vi "手绘波形子VI.vi"() -> (0 "输出的波形":waveform(dbl)(graph), 1 "最小值":dbl format="%#_3g", 2 "最大值":dbl format="%#_3g", 3 "频率":dbl)   [LabVIEW 2017]
uses:
  <vilib>/gmath/NI_Gmath.lvlib
panel:
  in  "选项卡控件":enum32{"手绘和参数设置", "输出的波形图", "使用说明"}(tab)
  out "绘 图 区":cluster{dbl, dbl}[](graph)
  in  "绘图完成":bool
  in  "时间长度":dbl=0.1
  in  "幅值":dbl=1.0
  # "手 绘 波 形"
  # "s"
  # "Hz"
  # "说明：\n1、鼠标在画板上单击并从左到右拖动，绘出所需的波形图；\n2、鼠标松开，鼠标单击绘图完成，自动生成所绘制的波形并退出此绘图界面；\n3、如果在上述绘图过程中，想重新绘制，可以点击幅值或者时间长度\n，只要其值发生改变，绘图区会自动清零."
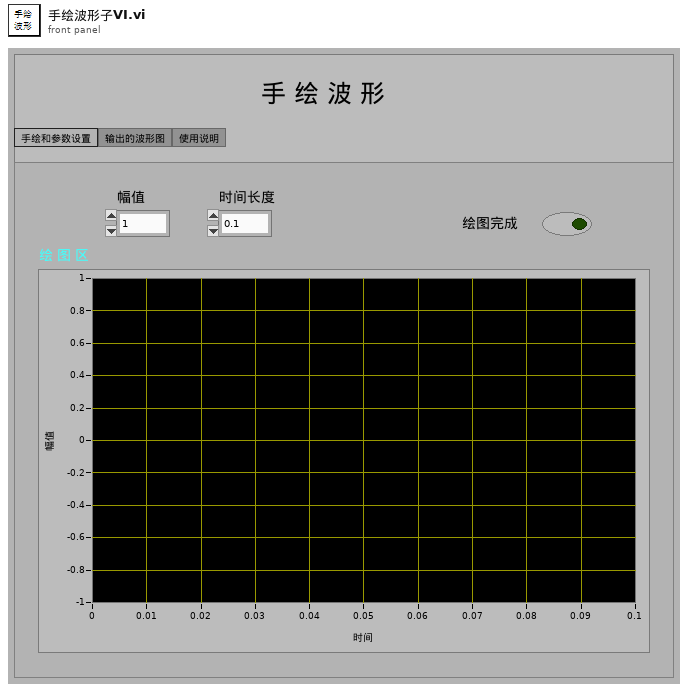
[diagram p1: front panel]
types:
  T1 = enum8{"Enabled", "Disabled", "Disabled and Grayed Out"}
  T2 = typedef "LVPoint32TypeDef.ctl" = cluster{"Horizontal":i32, "Vertical":i32}
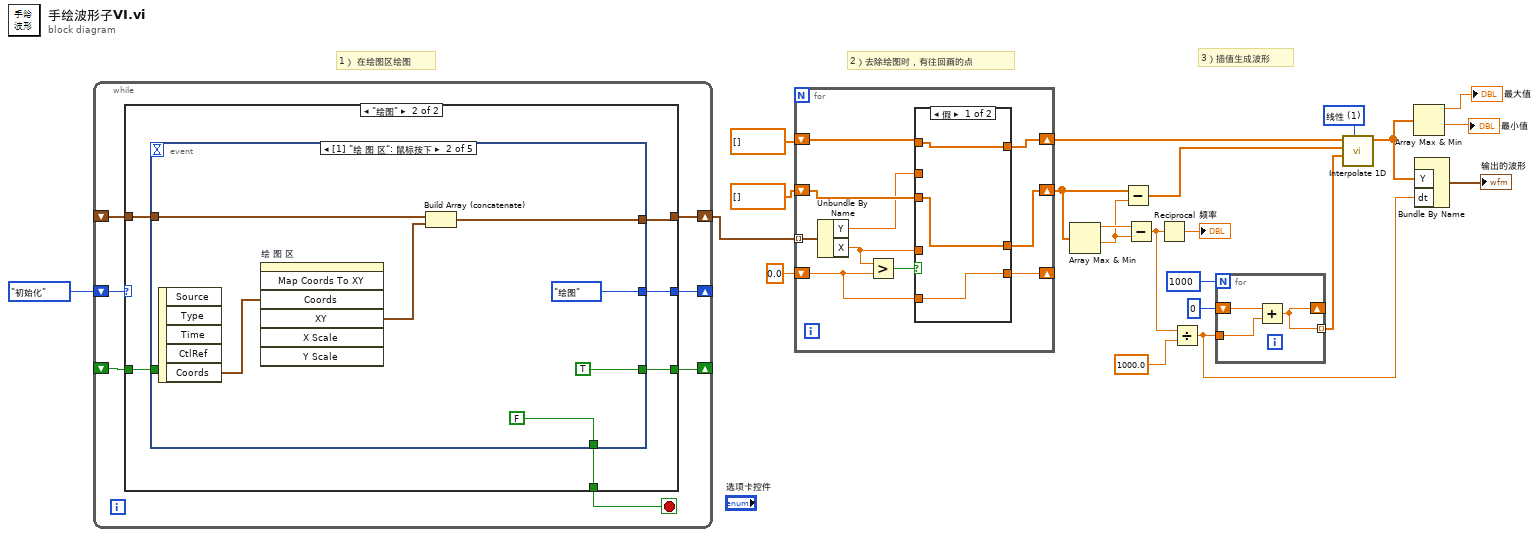
[diagram p0: block diagram]
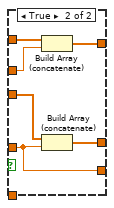
[diagram p2: hidden frame]
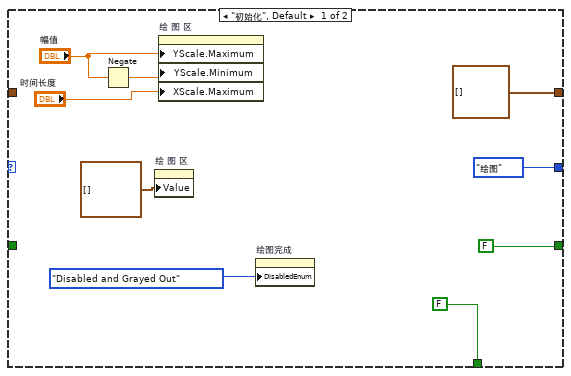
[diagram p3: hidden frame]
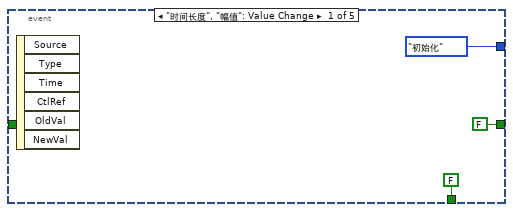
[diagram p4: hidden frame]
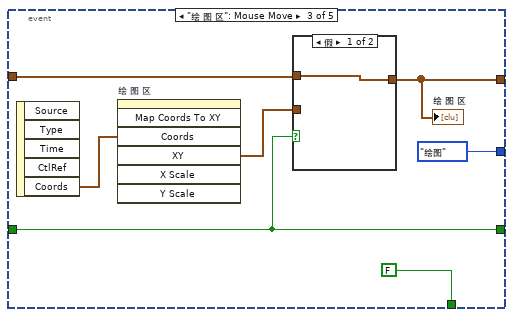
[diagram p5: hidden frame]
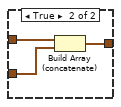
[diagram p6: hidden frame]
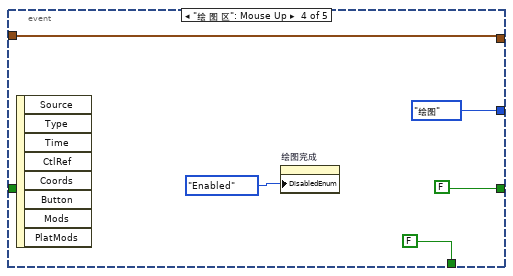
[diagram p7: hidden frame]
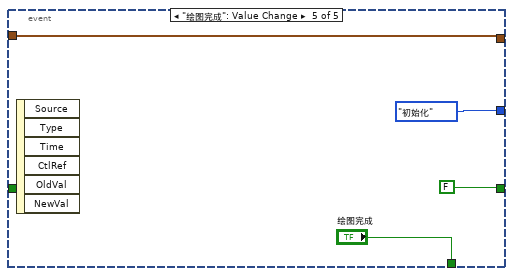
[diagram p8: hidden frame]
diagram:
  w14 = 1 items=["最近", "线性", "样条", "cubic Hermite", "拉格朗日"] ("method")
  # "3）插值生成波形"
  # "2）去除绘图时，有往回画的点"
  # "1） 在绘图区绘图"
  n1 = while {
    shift-right: [w29] -> w22
    shift-left: _ -> [w28]
    shift-right: [w23] -> _
    shift-left: enum16{"初始化", "绘图"}."初始化" -> [w27]
    shift-right: [w26] -> _
    shift-left: _ -> [w25]
    stop <- w24 stop-if-true
    n2 = case shown="\"绘图\"" w27 {
      tunnel: [cluster{"X":dbl, "Y":dbl}[] [] w44] -> w29
      tunnel: w28 -> [_ w43]
      tunnel: [FALSE ("press") w42] -> w26
      tunnel: w25 -> [_ w41]
      tunnel: [FALSE w40] -> w24
      tunnel: [enum16{"初始化", "绘图"}."绘图" w39] -> w23
      frame "初始化", Default {
        n3 = Negate(x="幅值") -> (-x=w37:dbl)
        n4 = property on="绘 图 区" class="XYGraph (严格)"("Value"=cluster{dbl, dbl}[] [] ("绘 图 区")) -> ()  [unwired: 2 in, 2 out]
        n5 = property on="绘 图 区" class="XYGraph (严格)"("YScale.Maximum"="幅值", "YScale.Minimum"=w37, "XScale.Maximum"="时间长度") -> ()  [unwired: 2 in, 2 out]
        n6 = property on="绘图完成" class="Bool"("DisabledEnum"=T1."Disabled and Grayed Out" ("禁用")) -> ()  [unwired: 2 in, 2 out]
      }
      frame "绘图" {
        n7 = event shown="[1] \"绘 图 区\": 鼠标按下" {
          selector: _ -> [_ _ _ _ _]
          dyn-events: _ -> [_ _ _ _ _]
          timeout: _ -> [_ _ _ _ _]
          tunnel: w43 -> [_ w53 w60 w70 w73]
          tunnel: [_ w51 w58 w70 w73] -> w44
          tunnel: [FALSE ("press") TRUE ("press") w57 FALSE ("press") FALSE ("press")] -> w42
          tunnel: w41 -> [_ _ w57 _ _]
          tunnel: [FALSE ("绘图完成") FALSE FALSE FALSE "绘图完成"] -> w40
          tunnel: [enum16{"初始化", "绘图"}."初始化" enum16{"初始化", "绘图"}."绘图" enum16{"初始化", "绘图"}."绘图" enum16{"初始化", "绘图"}."绘图" enum16{"初始化", "绘图"}."初始化"] -> w39
          event "时间长度", "幅值": Value Change {
            n8 = event-data() -> ()  [unwired: 1 in, 6 out]
          }
          event "绘 图 区": Mouse Down {
            n9 = event-data() -> ("Coords"=w54:T2)  [unwired: 1 in, 4 out]
            n10 = invoke on="绘 图 区" class="XYGraph (严格)" method="Map Coords To XY"("Coords"=w54) -> ("XY"=w52:cluster{"X":dbl, "Y":dbl})  [unwired: 6 in, 6 out]
            n11 = Build Array (concatenate)(w53, w52) -> (w51:cluster{"X":dbl, "Y":dbl}[])
          }
          event "绘 图 区": Mouse Move {
            n12 = event-data() -> ("Coords"=w61:T2)  [unwired: 1 in, 4 out]
            n13 = invoke on="绘 图 区" class="XYGraph (严格)" method="Map Coords To XY"("Coords"=w61) -> ("XY"=w59:cluster{"X":dbl, "Y":dbl})  [unwired: 6 in, 6 out]
            n14 = case shown="假" w57 {
              tunnel: w60 -> [w62 w65]
              tunnel: w59 -> [_ w64]
              tunnel: [w62 w63] -> w58
              frame False {
              }
              frame True {
                n15 = Build Array (concatenate)(w65, w64) -> (w63:cluster{"X":dbl, "Y":dbl}[])
              }
            }
            "绘 图 区" <- w58
          }
          event "绘 图 区": Mouse Up {
            n16 = event-data() -> ()  [unwired: 1 in, 8 out]
            n17 = property on="绘图完成" class="Bool"("DisabledEnum"=T1."Enabled" ("禁用")) -> ()  [unwired: 2 in, 2 out]
          }
          event "绘图完成": Value Change {
            n18 = event-data() -> ()  [unwired: 1 in, 6 out]
          }
        }
      }
    }
  }
  n19 = for {
    tunnel: w22 -> [w83] mode=indexing
    shift-right: [w80] -> w8
    shift-left: dbl[] [] -> [w82]
    shift-right: [w81] -> w2
    shift-left: dbl[] [] -> [w78]
    shift-right: [w79] -> _
    shift-left: 0.0 ("X") -> [w75]
    n20 = Unbundle By Name(w83) -> ("Y"=w76:dbl, "X"=w77:dbl)
    n21 = Greater?(x=w77, y=w75) -> (0:w84:bool)
    n22 = case shown="假" w84 {
      tunnel: w77 -> [_ w88]
      tunnel: w82 -> [w86 w90]
      tunnel: w76 -> [_ w91]
      tunnel: w78 -> [w87 w93]
      tunnel: [w87 w92] -> w81
      tunnel: [w86 w89] -> w80
      tunnel: [w85 w88] -> w79
      tunnel: w75 -> [w85 _]
      frame False {
      }
      frame True {
        n23 = Build Array (concatenate)(w93, w91) -> (w92:dbl[])
        n24 = Build Array (concatenate)(w90, w88) -> (w89:dbl[])
      }
    }
  }
  n25 = Array Max & Min(array=w8) -> (max value=w10:dbl, min value=w9:dbl)  [unwired: 2 out]
  n26 = Subtract(x=w8, y=w9) -> (x-y=w5:dbl[])
  n27 = Subtract(x=w10, y=w9) -> (x-y=w4:dbl)
  n28 = Reciprocal(x=w4) -> (1/x=→"频率":dbl)
  n29 = Divide(x=w4, y=1000.0) -> (x/y=w3:dbl)
  n30 = for {
    N: 1000 -> [_]
    shift-right: [w94] -> _
    shift-left: 0 -> [w95]
    tunnel: w3 -> [w96]
    tunnel: [w94] -> w6 mode=indexing
    n31 = Add(x=w95, y=w96) -> (x+y=w94:dbl)
  }
  n32 = call <vilib>:"Interpolate 1D.vi"("method"=w14, "xi"=w6, "X"=w5, "Y"=w2) -> ("yi"=w13:dbl[])  [unwired: 5 in, 2 out]
  n33 = Array Max & Min(array=w13) -> (max value=→"最大值":dbl, min value=→"最小值":dbl)  [unwired: 2 out]
  n34 = Bundle By Name("Y"=w13, "dt"=w3) -> (→"输出的波形":waveform(dbl))  [unwired: 1 in]
